vi "GT Set Enc Pos.vi"(8 "error in (no error)":errorcluster caption="错误输入（无错误）", 9 "encPos":i32, 10 "encoder":i16, 11 "cardNum":i16) -> (0 "error out":errorcluster caption="错误输出", 3 "function return":i16)   [LabVIEW 2014, in "gts.lvlib"]
doc: "GT_API GT_SetEncPos(short cardNum,short encoder,long encPos);"
uses:
  gts.lvlib
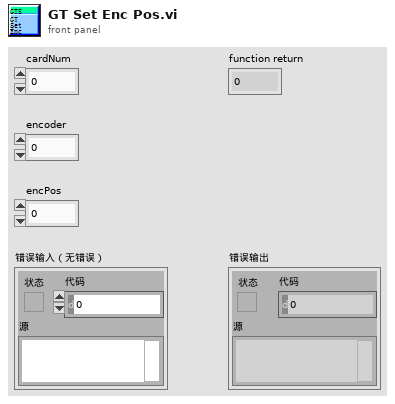
[diagram p1: front panel]
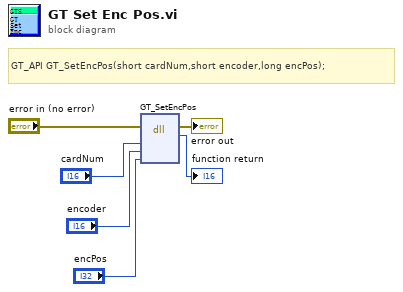
[diagram p0: block diagram]
diagram:
  # "GT_API GT_SetEncPos(short cardNum,short encoder,long encPos);"
  n1 = dll-call lib="PTH2habs D固高科技资料GTS控制卡GTS卡18年上半年资料dllVC32bit\nmulti_cardgts.*" fn="GT_SetEncPos"(error in="error in (no error)", "cardNum"="cardNum", "encoder"="encoder", "encPos"="encPos") -> (error out=→"error out":errorcluster, →"function return":i16)  [unwired: 5 in, 1 out]
